vi "Random bit generation.vi"(10 "total bits":i32) -> (2 "bit stream":u32[](array[numeric]))   [LabVIEW 2011]
uses:
  <vilib>/gmath/statdist.llb/Bernoulli Random.vi
  <vilib>/gmath/NI_Gmath.lvlib
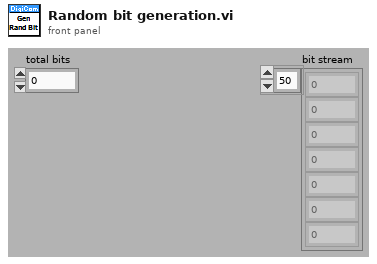
[diagram p1: front panel]
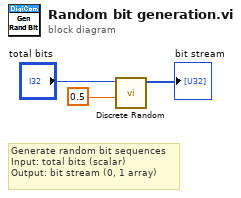
[diagram p0: block diagram]
diagram:
  # "Generate random bit sequences\nInput: total bits (scalar)\nOutput: bit stream (0, 1 array)"
  n1 = call-poly <vilib>:"Discrete Random.vi"("p"=0.5, "samples"="total bits") -> ("Bernoulli random numbers"=→"bit stream":u32[])  [unwired: 8 in, 1 out]
